vi "test_pathScalar.vi"(8 "error in (no error)":errorcluster) -> (0 "error out":errorcluster)   [LabVIEW 2013]
uses:
  run-tests/Run Test (Scalar Path).vi
  Caraya.lvlib
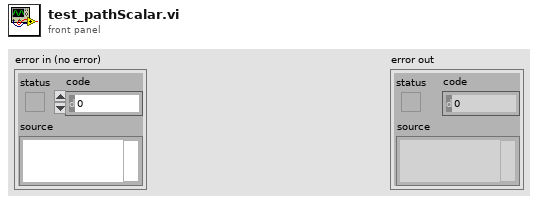
[diagram p1: front panel]
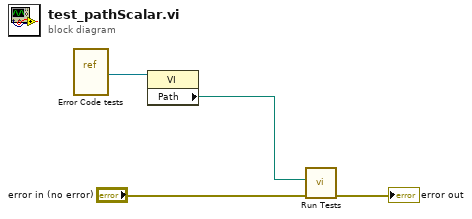
[diagram p0: block diagram]
diagram:
  n1 = vi-ref "Error Code tests.vi"() -> (w4:refnum<vi>)
  n2 = property class="VI"(reference=w4) -> ("Path"=w1:path)  [unwired: 1 in, 2 out]
  n3 = call-poly "Run Tests.vi"("error in"="error in (no error)", "Test Path"=w1) -> ("error out"=→"error out":errorcluster)  [unwired: 8 in, 1 out]
